vi "Close VI.vi"(10 "Log File Cluster":T1) -> (2 "State Ring":u16(ring) items=["Init VI", "Init Event Handlers", "Booting sequence", "Operational", "Emergency shutting down", "Shuting down", "Closing VI"])   [LabVIEW 2016]
uses:
  Log File Cluster.ctl
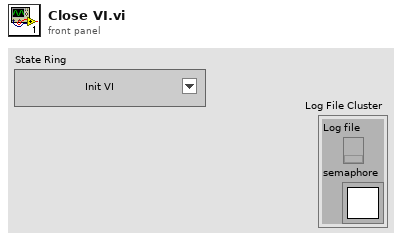
[diagram p1: front panel]
types:
  T1 = typedef "Log File Cluster.ctl" = cluster{"Log file":refnum<k34>, "semaphore":T2}
  T2 = typedef "Semaphore RefNum" = refnum<k1>
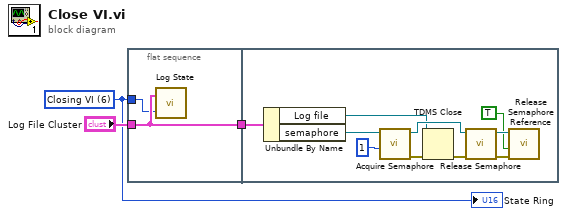
[diagram p0: block diagram]
diagram:
  w1 = u16 6 items=["Init VI", "Init Event Handlers", "Booting sequence", "Operational", "Emergency shutting down", "Shuting down", "Closing VI"] ("State Ring")
  n1 = flat-sequence {
    tunnel: "Log File Cluster" -> [w5]
    tunnel: [w5] -> w2
    tunnel: w1 -> [w4]
    tunnel: w2 -> [w7]
    frame #0 {
      n2 = call "Log State.vi"("State Ring"=w4, "Log File Cluster"=w5) -> ()  [unwired: 1 in]
    }
    frame #1 {
      n3 = Unbundle By Name(w7) -> ("Log file"=w6:refnum<k34>, "semaphore"=w15:T2)
      n4 = call <vilib>:"Acquire Semaphore.vi"("ms timeout (-1)"=1, "semaphore"=w15) -> ("error out"=w9:errorcluster, "semaphore out"=w13:T2)  [unwired: 3 in, 1 out]
      n5 = TDMS Close(8:w9, 11:w6) -> (0:w8:errorcluster)  [unwired: 1 out]
      n6 = call <vilib>:"Release Semaphore.vi"("error in (no error)"=w8, "semaphore"=w13) -> ("error out"=w11:errorcluster, "semaphore out"=w12:T2)  [unwired: 4 in]
      n7 = call <vilib>:"Release Semaphore Reference.vi"("error in (no error)"=w11, "force destroy? (F)"=TRUE, "semaphore"=w12) -> ()  [unwired: 7 in, 2 out]
    }
  }
  "State Ring" <- w1
